vi "Find Test Cases in LV XML.vi"(8 "error in (no error)":errorcluster, 11 "Project Path":path) -> (0 "error out":errorcluster, 2 "Test Class paths":path[](array[path]))   [LabVIEW 2020, in "Test Finder.lvclass"]
uses:
  Test Finder.lvclass
  Test Finder.lvclass/Test Finder.ctl
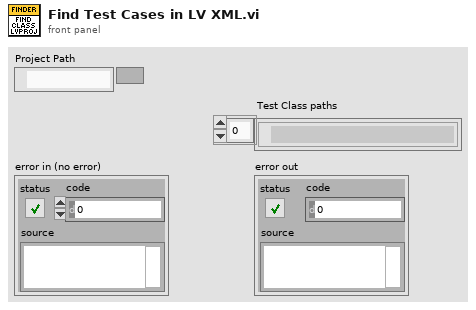
[diagram p1: front panel]
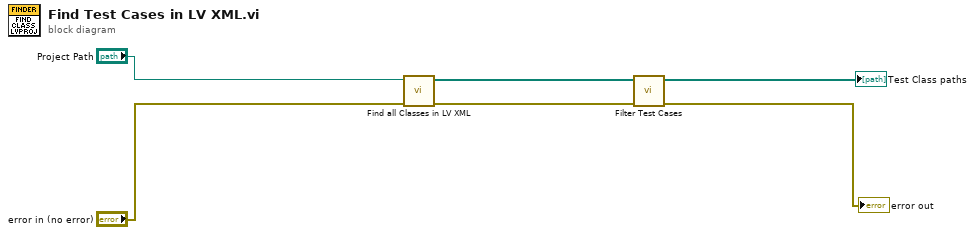
[diagram p0: block diagram]
diagram:
  n1 = call "Find all Classes in LV XML.vi"("error in (no error)"="error in (no error)", "Project Path"="Project Path") -> ("error out"=w1:errorcluster, "Class Paths"=w4:path[])  [unwired: 8 in]
  n2 = call "Filter Test Cases.vi"("error in (no error)"=w1, "Classes to Filter"=w4) -> ("error out"=→"error out":errorcluster, "Filtered Classes"=→"Test Class paths":path[])  [unwired: 8 in]
